vi "Populate Tests.vi"(8 "error in (no error)":errorcluster, 10 "List of Tests":string[](array[string]), 11 "Test Tree In":refnum<class "Test Result Tree V2.lvclass">) -> (0 "error out":errorcluster, 3 "Test Tree Out":refnum<class "Test Result Tree V2.lvclass">)   [LabVIEW 2020, in "Test Result Tree V2.lvclass"]
uses:
  Test Result Tree V2.lvclass
  C:/Git/astemes-lunit/source/Rewrite Project/Test Tree/Test Tree.lvclass
  Test Tree/Test Tree.lvclass/Test Tree.ctl
  <vilib>/Utility/miscctls.llb/LVMapReplaceAction.ctl
  Test Tree/Test Tree.lvclass
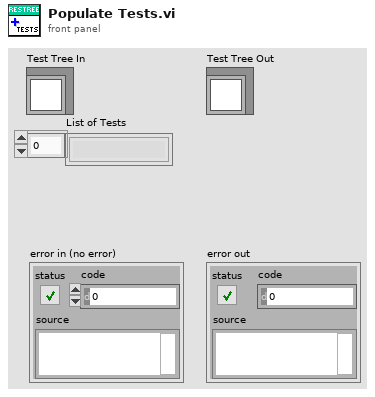
[diagram p1: front panel]
types:
  T1 = map{string, cluster{"Left Cell String":string, "Child Text":string[], "Item Indent":i32, "Child Only?":bool, "Glyph Index":i32}}
  T2 = typedef "LVMapReplaceAction.ctl" = enum32{"Modify Entry only if found", "Add or Modify Entry", "Delete Entry"}
  T3 = cluster{"Left Cell String":string, "Child Text":string[], "Item Indent":i32, "Child Only?":bool, "Glyph Index":i32}
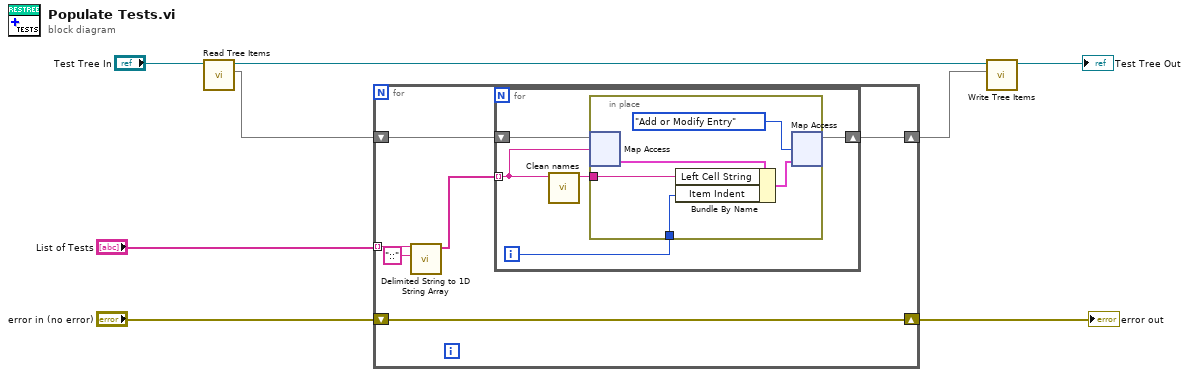
[diagram p0: block diagram]
diagram:
  n1 = call "Read Tree Items.vi"("Test Tree In"="Test Tree In") -> ("Tree Items"=w2:T1, "Test Tree Out"=w3:refnum<class "Test Result Tree V2.lvclass">)  [unwired: 9 in]
  n2 = for {
    shift-right: [w14] -> w7
    shift-left: "error in (no error)" -> [w14]
    shift-right: [w12] -> w5
    shift-left: w2 -> [w13]
    tunnel: "List of Tests" -> [w11] mode=indexing
    n3 = call <vilib>:"Delimited String to 1D String Array.vi"("delimiter"="::", "delimited string"=w11) -> ("string array"=w9:string[])  [unwired: 9 in]
    n4 = for {
      tunnel: w9 -> [w17] mode=indexing
      shift-right: [w18] -> w12
      shift-left: w13 -> [w19]
      i -> [w15]
      n5 = call "Clean names.vi"("Name with extension"=w17) -> ("Name without extension"=w16:string)  [unwired: 10 in]
      n6 = in-place {
        in-place-border: w16 -> [w23]
        in-place-border: w15 -> [w20]
        n7 = in-place-map #1(w19, w17) -> (w24:T3)  [unwired: 1 in, 1 out]
        n8 = Bundle By Name(cluster=w24, "Left Cell String"=w23, "Item Indent"=w20) -> (w22:T3)
        n9 = in-place-map #1(w22, LVMapReplaceAction."Add or Modify Entry" ("action")) -> (w18:T1)  [unwired: 2 out]
      }
    }
  }
  "error out" <- w7
  n10 = call "Write Tree Items.vi"("Tree Items"=w5, "Test Tree In"=w3) -> ("Test Tree Out"=→"Test Tree Out":refnum<class "Test Result Tree V2.lvclass">)  [unwired: 9 in]
